vi "Gesha_UTS1.vi"() -> ()   [LabVIEW 2020]
panel:
  out "WARNING":bool
  in  "HIGH Limit":dbl(slide) scale=0.0..100.0
  in  "LOW Limit":dbl(slide) scale=0.0..100.0
  in  "Operator":string
  out "Waveform Chart":T1(graph)
  out "START/STOP":bool
  in  "STOP":bool
  in  "START/STOP":bool
  in  "C   or   F":bool
  in  "Filename":path
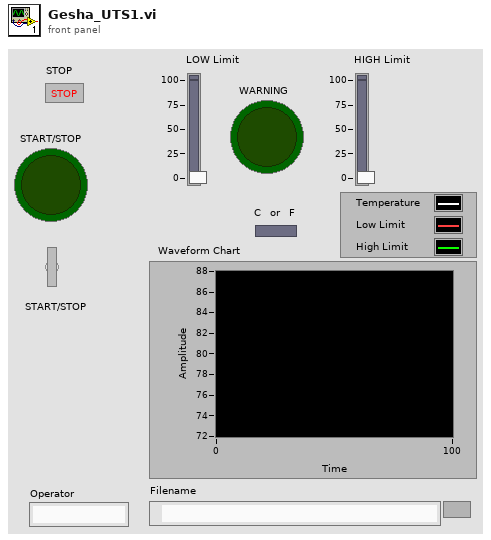
[diagram p1: front panel]
types:
  T1 = cluster{"Temperature (deg F)":dbl, "LOW Limit":dbl, "HIGH Limit":dbl}
  T2 = enum16{"open", "replace", "create", "open or create", "replace or create", "replace or create with confirmation"}
  T3 = cluster{"Y":dbl, "LOW Limit":dbl, "HIGH Limit":dbl}
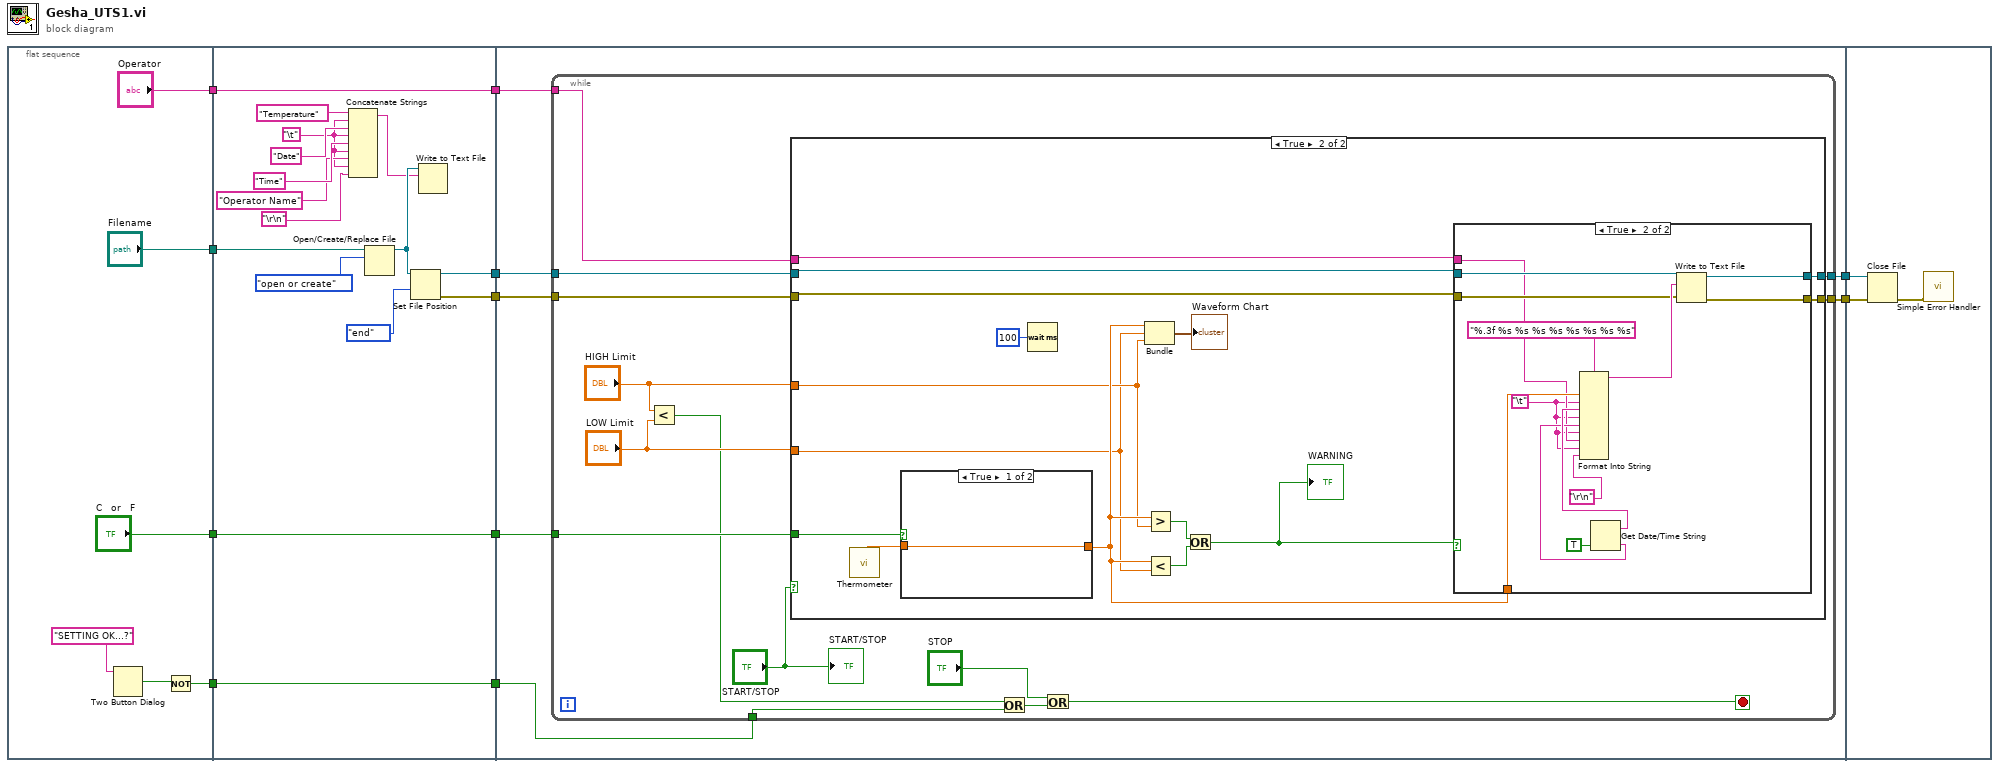
[diagram p0: block diagram]
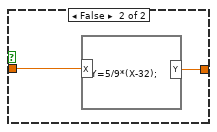
[diagram p4: hidden frame]
diagram:
  n1 = flat-sequence {
    tunnel: ["Filename"] -> w11
    tunnel: ["C   or   F"] -> w9
    tunnel: [w13] -> w7
    tunnel: ["Operator"] -> w1
    tunnel: w11 -> [w33]
    tunnel: [w31] -> w10
    tunnel: w9 -> [w31]
    tunnel: [w30] -> w8
    tunnel: w7 -> [w30]
    tunnel: [w29] -> w6
    tunnel: [w28] -> w5
    tunnel: [w25] -> w2
    tunnel: w1 -> [w25]
    tunnel: w10 -> [w40]
    tunnel: w8 -> [w39]
    tunnel: w6 -> [w38]
    tunnel: w5 -> [w37]
    tunnel: [w36] -> w4
    tunnel: [w35] -> w3
    tunnel: w2 -> [w34]
    tunnel: w4 -> [w92]
    tunnel: w3 -> [w91]
    frame #0 {
      n2 = Two Button Dialog(message="SETTING OK...?") -> (T button?=w14:bool)  [unwired: 2 in]
      n3 = Not(x=w14) -> (.not. x?=w13:bool)
    }
    frame #1 {
      w18 = "\t"
      n4 = Concatenate Strings("Temperature" ("string"), w18, "Date" ("string"), w18, "Time" ("string"), w18, "Operator Name" ("string"), w18, "\r\n") -> (w24:string)
      n5 = Open/Create/Replace File(file path (use dialog)=w33, operation (0:open)=T2."open or create") -> (refnum out=w27:refnum<file>)  [unwired: 4 in, 2 out]
      n6 = Set File Position(refnum=w27, from (0:start)=enum16{"start", "end", "current"}."end") -> (refnum out=w29:refnum<file>, error out=w28:errorcluster)  [unwired: 2 in]
      n7 = Write to Text File(file (use dialog)=w27, text=w24) -> ()  [unwired: 2 in, 3 out]
    }
    frame #2 {
      n8 = while {
        tunnel: w40 -> [w54]
        tunnel: w39 -> [w53]
        tunnel: w38 -> [w52]
        tunnel: w37 -> [w51]
        tunnel: [w50] -> w36
        tunnel: [w49] -> w35
        tunnel: w34 -> [w48]
        stop <- w45 stop-if-true
        n9 = Less?(x="HIGH Limit", y="LOW Limit") -> (x < y?=w42:bool)
        n10 = case shown="True" "START/STOP" {
          tunnel: w54 -> [_ w71]
          tunnel: w52 -> [w56 w66]
          tunnel: w51 -> [w55 w65]
          tunnel: [w56 w64] -> w50
          tunnel: [w55 w63] -> w49
          tunnel: w48 -> [_ w62]
          tunnel: "HIGH Limit" -> [_ w59]
          tunnel: "LOW Limit" -> [_ w58]
          frame False {
          }
          frame True {
            n11 = call "Thermometer.vi"() -> ("Temperature (deg F)"=w60:dbl)  [unwired: 1 in]
            n12 = case shown="True" w71 {
              tunnel: w60 -> [w87 w89]
              tunnel: [w87 w88] -> w61
              frame True {
              }
              frame False {
                n13 = formula code="Y=5/9*(X-32);"("X"=w89) -> ("Y"=w88:dbl)
              }
            }
            n14 = Wait (ms)(milliseconds to wait=u32 100) -> ()  [unwired: 1 out]
            n15 = Bundle("Y"=w61, "LOW Limit"=w58, "HIGH Limit"=w59) -> (→"Waveform Chart":T3)  [unwired: 1 in]
            n16 = Greater?(x=w61, y=w59) -> (0:w70:bool)
            n17 = Less?(x=w61, y=w58) -> (x < y?=w69:bool)
            n18 = Or(x=w70, y=w69) -> (x .or. y?=w57:bool)
            "WARNING" <- w57
            n19 = case shown="True" w57 {
              tunnel: w61 -> [_ w85]
              tunnel: w66 -> [w72 w83]
              tunnel: w65 -> [w73 w82]
              tunnel: [w72 w81] -> w64
              tunnel: [w73 w80] -> w63
              tunnel: w62 -> [_ w75]
              frame False {
              }
              frame True {
                w74 = "\t"
                n20 = Get Date/Time String(want seconds? (F)=TRUE) -> (date string=w78:string, time string=w77:string)  [unwired: 2 in]
                n21 = Format Into String "Format Into String"(format string="%.3f %s %s %s %s %s %s %s %s", w85, w74, w78, w74, w77, w74, w75, w74, "\r\n") -> (resulting string=w84:string)  [unwired: 2 in, 1 out]
                n22 = Write to Text File(file (use dialog)=w83, text=w84, error in=w82) -> (refnum out=w81:refnum<file>, error out=w80:errorcluster)  [unwired: 1 in, 1 out]
              }
            }
          }
        }
        n23 = Or(x=w42, y=w53) -> (x .or. y?=w46:bool)
        n24 = Or(x="STOP", y=w46) -> (x .or. y?=w45:bool)
        "START/STOP" <- "START/STOP"
      }
    }
    frame #3 {
      n25 = Close File(refnum=w92, error in=w91) -> (error out=w90:errorcluster)  [unwired: 1 out]
      n26 = call <vilib>:"Simple Error Handler.vi"("error in (no error)"=w90) -> ()  [unwired: 4 in, 5 out]
    }
  }
